vi "clarke.vi"() -> ()   [LabVIEW 2015]
uses:
  <vilib>/Analysis/baseanly.llb/Mean (DBL).vi
  <vilib>/Analysis/NI_AALBase.lvlib
panel:
  out "SGL error max":dbl
  out "SGL error mean":dbl format="%0.2f"
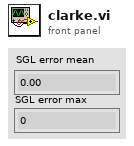
[diagram p1: front panel]
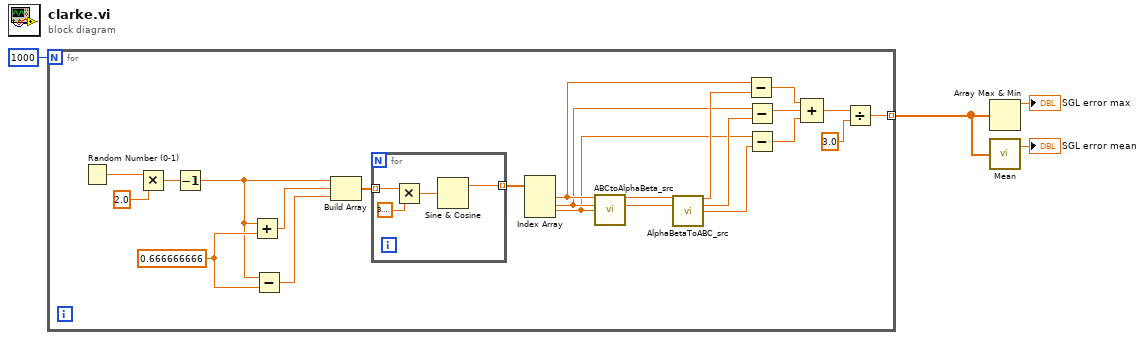
[diagram p0: block diagram]
diagram:
  n1 = for {
    N: 1000 -> [_]
    tunnel: [w11] -> w4 mode=indexing
    w25 = 0.666666666
    n2 = Random Number (0-1)() -> (number: 0 to 1=w7:dbl)
    n3 = Multiply(x=w7, y=2.0) -> (x*y=w26:dbl)
    n4 = Decrement(x=w26) -> (x-1=w17:dbl)
    n5 = Add(x=w17, y=w25) -> (x+y=w18:dbl)
    n6 = Subtract(x=w17, y=w25) -> (x-y=w19:dbl)
    n7 = Build Array(w17, w18, w19) -> (w24:dbl[])
    n8 = for {
      tunnel: w24 -> [w31] mode=indexing
      tunnel: [w28] -> w23 mode=indexing
      n9 = Multiply(x=w31, y=3.141592653589793) -> (x*y=w29:dbl)
      n10 = Sine & Cosine(0:w29) -> (1:w28:dbl)  [unwired: 1 out]
    }
    n11 = Index Array(array=w23) -> (element #1=w10:dbl, element #2=w9:dbl, element #3=w8:dbl)  [unwired: 3 in]
    n12 = call "ABCtoAlphaBeta_src.vi"("A"=w10, "B"=w9, "C"=w8) -> ("alpha"=w6:sgl, "beta"=w5:sgl)  [unwired: 11 in]
    n13 = call "AlphaBetaToABC_src.vi"("alpha"=w6, "beta"=w5) -> ("A"=w22:sgl, "B"=w20:sgl, "C"=w21:sgl)  [unwired: 11 in]
    n14 = Subtract(x=w10, y=w22) -> (x-y=w16:dbl)
    n15 = Subtract(x=w9, y=w20) -> (x-y=w15:dbl)
    n16 = Subtract(x=w8, y=w21) -> (x-y=w14:dbl)
    n17 = Compound Arithmetic op=ADD(w16, w15, w14) -> (w13:dbl)
    n18 = Divide(x=w13, y=3.0) -> (x/y=w11:dbl)
  }
  n19 = Array Max & Min(array=w4) -> (max value=→"SGL error max":dbl)  [unwired: 3 out]
  n20 = call-poly <vilib>:"Mean.vi"("X"=w4) -> ("mean"=→"SGL error mean":dbl)  [unwired: 1 out]
